vi "2-ReadAllFiles.vi"(8 "error in (no error)":errorcluster, 11 "AllControls IN":T1) -> (0 "error out":errorcluster, 3 "AllControls Out":T1)   [LabVIEW 2017]
uses:
  Ctrls/AllControls.ctl
  <vilib>/Utility/miscctls.llb/LVRowAndColumnTypeDef.ctl
  Ctrls/Position Config.ctl
  Ctrls/TesterInfo.ctl
  Ctrls/HD Config.ctl
  <vilib>/Utility/file.llb/Read Delimited Spreadsheet (string).vi
  ComVIS/Files/Ini/ReadIniFiles_ByVarient.vi
  <vilib>/regexp/Match Regular Expression.xnode
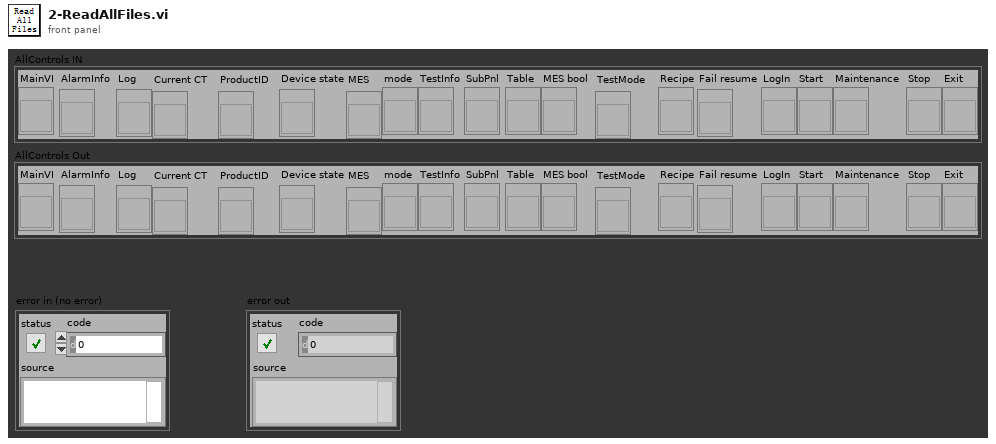
[diagram p1: front panel]
types:
  T1 = typedef "AllControls.ctl" = cluster{"MainVI":refnum<vi>, "AlarmInfo":refnum<vi>, "Log":refnum<vi>, "Current CT":refnum<vi>, "ProductID":refnum<vi>, "Device state":refnum<vi>, "MES":refnum<vi>, "mode":refnum<vi>, "TestInfo":refnum<vi>, "SubPnl":refnum<vi>, "Table":refnum<vi>, "MES bool":refnum<vi>, "TestMode":refnum<vi>, "Recipe":refnum<vi>, "Fail resume":refnum<vi>, "LogIn":refnum<vi>, "Start":refnum<vi>, "Maintenance":refnum<vi>, "Stop":refnum<vi>, "Exit":refnum<vi>}
  T2 = typedef "HD Config.ctl" = cluster{" PC":cluster{"PC Address":u8[], "PC Port":i32}, "FCO":cluster{"COM":refnum<visa-resource-name>, "Baudrate":u32}, "DC Power ":cluster{"COM":refnum<visa-resource-name>, "Baudrate":u32}, "PW3336":cluster{"COM":refnum<visa-resource-name>, "Baudrate":u32}, "Lefoo":cluster{"COM":refnum<visa-resource-name>, "Baudrate":u32}, "Tempt&Hum":cluster{"COM":refnum<visa-resource-name>, "Baudrate":u32}, "DIPC":cluster{"COM":refnum<visa-resource-name>}, "Daemon":cluster{"IP Address":string, "Port":u16, "Retry":u16}, "NFC_Cmd":cluster{"COM":refnum<visa-resource-name>, "Baudrate":u32}, "Fail_resume_mode":bool, "GRR":bool, "NFC _Serial":cluster{"COM":refnum<visa-resource-name>, "Baudrate":u32}}
  T3 = typedef "TesterInfo.ctl" = cluster{"Station Name":string, "Station Code":string, "ES NO.":string, "Tester ID":string, "PassMark Revision":string, "Rig ID":string, "682_Tool_Repeat":string, "Project Name":string, "FFTesterPath":path, "Enable_User":bool, "Mode":enum16{"682"}, "Fail_resume_mode":bool}
  T4 = typedef "Position Config.ctl" = cluster{"Black":dbl, "White":dbl, "Black1":dbl, "White1":dbl}
  T5 = typedef "LVRowAndColumnTypeDef.ctl" = cluster{"Row":i32, "Column":i32}
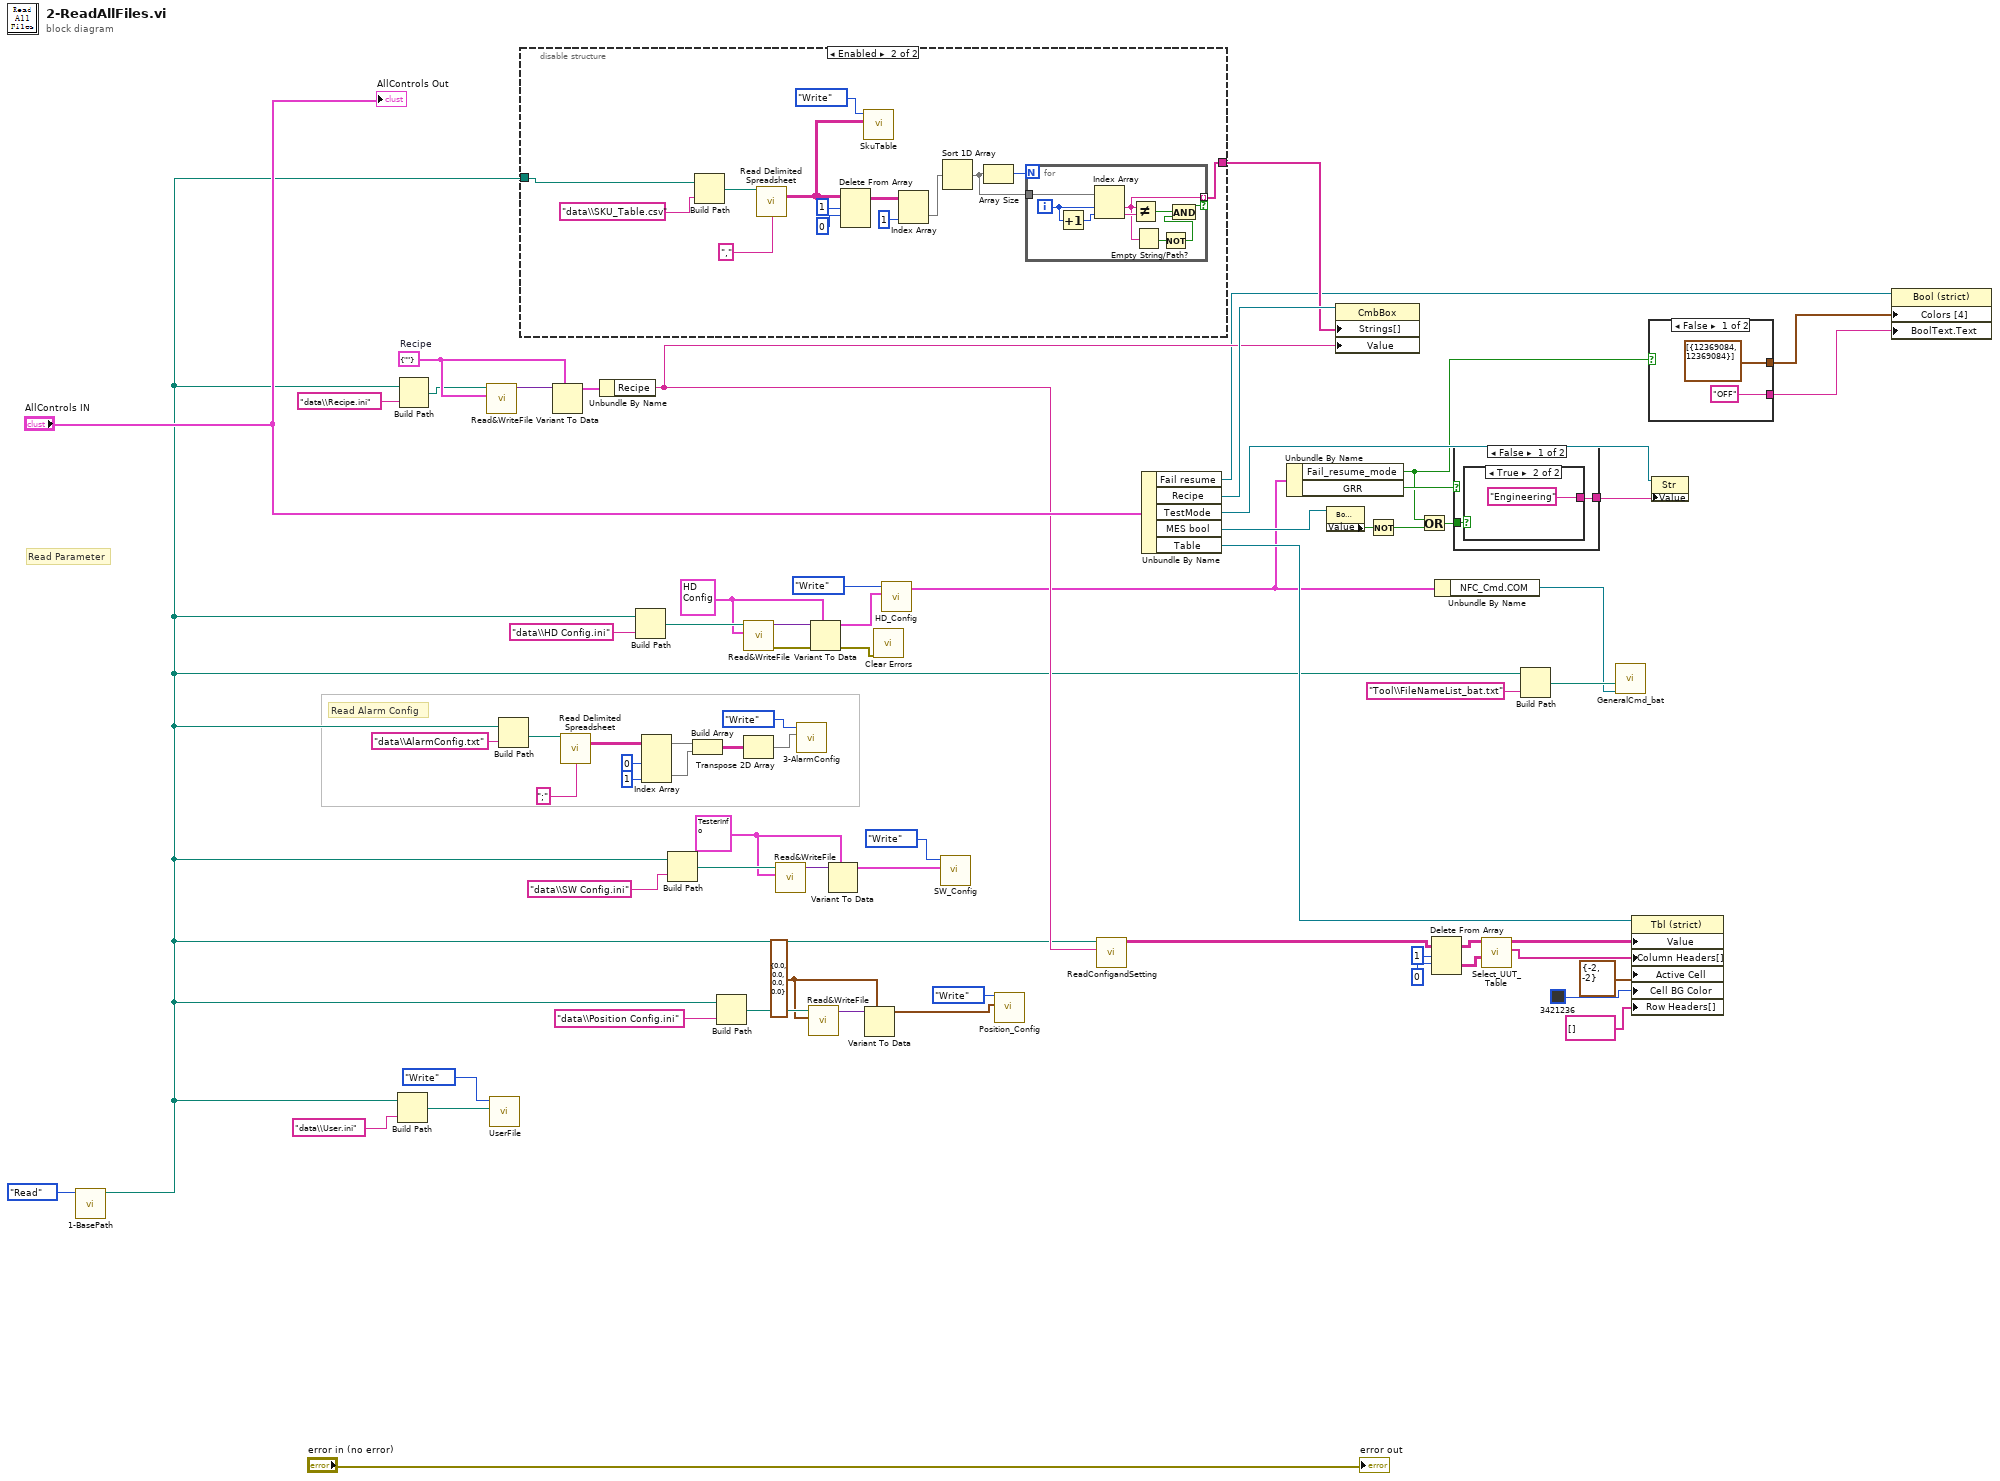
[diagram p0: block diagram]
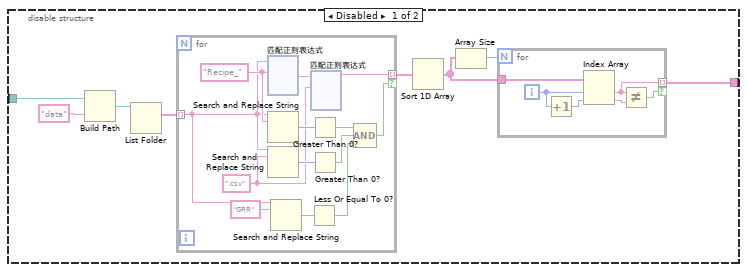
[diagram p2: hidden frame]
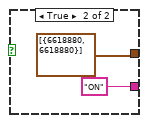
[diagram p3: hidden frame]
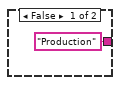
[diagram p4: hidden frame]
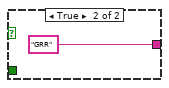
[diagram p5: hidden frame]
diagram:
  w15 = cluster{"Recipe":string} {"Recipe"=""}  # Recipe
  w26 = T2 {" PC"={"PC Address"=[], "PC Port"=0}, "FCO"={"COM"="", "Baudrate"=0}, "DC Power "={"COM"="", "Baudrate"=0}, "PW3336"={"COM"="", "Baudrate"=0}, "Lefoo"={"COM"="", "Baudrate"=0}, "Tempt&Hum"={"COM"="", "Baudrate"=0}, "DIPC"={"COM"=""}, "Daemon"={"IP Address"="", "Port"=0, "Retry"=0}, "NFC_Cmd"={"COM"="", "Baudrate"=0}, "Fail_resume_mode"=FALSE, "GRR"=FALSE, "NFC _Serial"={"COM"="", "Baudrate"=0}} ("HD Config")
  w27 = T3 {"Station Name"="", "Station Code"="", "ES NO."="", "Tester ID"="", "PassMark Revision"="", "Rig ID"="", "682_Tool_Repeat"="", "Project Name"="", "FFTesterPath"=path "", "Enable_User"=FALSE, "Mode"=enum."682", "Fail_resume_mode"=FALSE} ("TesterInfo")
  w30 = T4 {"Black"=0.0, "White"=0.0, "Black1"=0.0, "White1"=0.0} ("Position Config")
  # "Read Alarm Config"
  # "Read Parameter"
  n1 = call "1-BasePath.vi"("Step"=enum16{"Initial", "Write", "Read"}."Read") -> ("Path Out"=w1:path)  [unwired: 9 in, 1 out]
  n2 = Build Path(base path=w1, name or relative path="data\\User.ini") -> (appended path=w48:path)
  n3 = Build Path(base path=w1, name or relative path="data\\Recipe.ini") -> (appended path=w12:path)
  n4 = call-poly "Read&WriteFile.vi"("Varient"=w15, "path"=w12) -> ("DataOut"=w16:variant)  [unwired: 8 in, 1 out]
  n5 = call "UserFile.vi"("UserPath in"=w48, "Step"=enum16{"Initial", "Write", "Read"}."Write") -> ()  [unwired: 8 in, 2 out]
  n6 = Build Path(base path=w1, name or relative path="data\\AlarmConfig.txt") -> (appended path=w63:path)
  n7 = disable-structure shown="Enabled" {
    disable-tunnel: [w74 w330] -> w17
    disable-tunnel: w1 -> [w73 w337]
    frame Disabled {
      n8 = Build Path(base path=w73, name or relative path="data") -> (appended path=w79:path)
      n9 = List Folder(path=w79) -> (filenames=w78:string[])  [unwired: 3 in, 3 out]
      n10 = for {
        tunnel: w78 -> [w90] mode=indexing
        tunnel: [w91] -> w77 mode=indexing if=w97
        w92 = ".csv" ("搜索字符串")
        w94 = "Recipe_" ("搜索字符串")
        n11 = xnode "匹配正则表达式"("输入字符串"=w90, "正则表达式"=w94) -> ("匹配之后"=w93:string)  [unwired: 4 in, 4 out]
        n12 = Search and Replace String(input string=w90, search string=w94) -> (number of replacements=w99:i32)  [unwired: 6 in, 3 out]
        n13 = Search and Replace String(input string=w90, search string=w92) -> (number of replacements=w96:i32)  [unwired: 6 in, 3 out]
        n14 = Search and Replace String(input string=w90, search string="GRR" ("搜索字符串")) -> (number of replacements=w88:i32)  [unwired: 6 in, 3 out]
        n15 = Less Or Equal To 0?(x=w88) -> (x <= 0?=w87:bool)
        n16 = Greater Than 0?(x=w99) -> (x > 0?=w98:bool)
        n17 = Greater Than 0?(x=w96) -> (x > 0?=w95:bool)
        n18 = xnode "匹配正则表达式"("输入字符串"=w93, "正则表达式"=w92) -> ("匹配之前"=w91:string)  [unwired: 4 in, 4 out]
        n19 = Compound Arithmetic op=AND ("复合运算")(w98, w95, w87) -> (w97:bool)
      }
      n20 = Sort 1D Array(array=w77) -> (sorted array=w75:string[])
      n21 = Array Size(array=w75) -> (size(s)=w76:i32)
      n22 = for {
        N: w76 -> [_]
        tunnel: w75 -> [w86]
        tunnel: [w82] -> w74 mode=indexing if=w85
        i -> [w84]
        n23 = Increment(x=w84) -> (x+1=w83:i32)
        n24 = Index Array(array=w86, index #1=w84, index #2=w83) -> (element #1=w82:string, element #2=w81:string)
        n25 = Not Equal?(x=w82, y=w81) -> (x != y?=w85:bool)
      }
    }
    frame Enabled {
      n26 = Build Path(base path=w337, name or relative path="data\\SKU_Table.csv") -> (appended path=w341:path)
      n27 = call-poly <vilib>:"Read Delimited Spreadsheet.vi"("file path (dialog if empty)"=w341, "delimiter (\\t)"="," ("delimiter (\\t)")) -> ("all rows"=w336:string[][])  [unwired: 8 in, 5 out]
      n28 = Delete From Array(array=w336, length=1 ("长度"), index (row)=0 ("索引 (行)")) -> (array with subset deleted=w333:string[][])  [unwired: 1 in, 1 out]
      n29 = call "SkuTable.vi"("Tabledata in"=w336, "Step"=enum16{"Initial", "Write", "Read"}."Write") -> ()  [unwired: 8 in, 2 out]
      n30 = Index Array(array=w333, index (col)=1 ("禁用的索引 (列)")) -> (element=w328:string[])  [unwired: 1 in]
      n31 = Sort 1D Array(array=w328) -> (sorted array=w329:string[])
      n32 = Array Size(array=w329) -> (size(s)=w331:i32)
      n33 = for {
        N: w331 -> [_]
        tunnel: w329 -> [w350]
        tunnel: [w345] -> w330 mode=indexing if=w343
        i -> [w348]
        n34 = Increment(x=w348) -> (x+1=w347:i32)
        n35 = Index Array(array=w350, index #1=w348, index #2=w347) -> (element #1=w345:string, element #2=w346:string)
        n36 = Not Equal?(x=w345, y=w346) -> (x != y?=w349:bool)
        n37 = Empty String/Path?(string/path=w345) -> (empty?=w344:bool)
        n38 = Not(x=w344) -> (.not. x?=w342:bool)
        n39 = And(x=w349, y=w342) -> (x .and. y?=w343:bool)
      }
    }
  }
  n40 = Variant To Data(type=w15, Variant=w16) -> (data=w14:cluster{"Recipe":string})  [unwired: 1 in, 1 out]
  n41 = call-poly <vilib>:"Read Delimited Spreadsheet.vi"("file path (dialog if empty)"=w63, "delimiter (\\t)"=";" ("delimiter (\\t)")) -> ("all rows"=w60:string[][])  [unwired: 8 in, 5 out]
  n42 = Unbundle By Name(w14) -> ("Recipe"=w11:string)
  n43 = Build Path(base path=w1, name or relative path="data\\HD Config.ini") -> (appended path=w68:path)
  n44 = Index Array(array=w60, index (col) #1=0 ("disabled index (col)"), index (col) #2=1 ("index (col)")) -> (element #1=w59:string[], element #2=w55:string[])  [unwired: 2 in]
  n45 = Build Path(base path=w1, name or relative path="data\\SW Config.ini") -> (appended path=w52:path)
  n46 = Build Array(w59, w55) -> (w56:string[][])
  n47 = Build Path(base path=w1, name or relative path="data\\Position Config.ini") -> (appended path=w33:path)
  n48 = call-poly "Read&WriteFile.vi"("Varient"=w26, "path"=w68) -> ("error out"=w66:errorcluster, "DataOut"=w67:variant)  [unwired: 8 in]
  n49 = Transpose 2D Array(2D array=w56) -> (transposed array=w54:string[][])
  n50 = call-poly "Read&WriteFile.vi"("Varient"=w27, "path"=w52) -> ("DataOut"=w50:variant)  [unwired: 8 in, 1 out]
  n51 = call "3-AlarmConfig.vi"("AlarmConfig In"=w54, "Step"=enum16{"Initial", "Write", "Read"}."Write") -> ()  [unwired: 8 in, 2 out]
  n52 = call-poly "Read&WriteFile.vi"("Varient"=w30, "path"=w33) -> ("DataOut"=w31:variant)  [unwired: 8 in, 1 out]
  n53 = Variant To Data(error in=w66, type=w26, Variant=w67) -> (data=w46:T2, error out=w65:errorcluster)
  n54 = Variant To Data(type=w27, Variant=w50) -> (data=w45:T3)  [unwired: 1 in, 1 out]
  n55 = Variant To Data(type=w30, Variant=w31) -> (data=w29:T4)  [unwired: 1 in, 1 out]
  n56 = call <vilib>:"Clear Errors.vi"("error in (no error)"=w65) -> ()  [unwired: 5 in, 2 out]
  n57 = call "HD_Config.vi"("HD Config in"=w46, "Step"=enum16{"Initial", "Write", "Read"}."Write") -> ("HD Config out"=w2:T2)  [unwired: 8 in, 1 out]
  n58 = call "SW_Config.vi"("SW Config In"=w45, "Step"=enum16{"Initial", "Write", "Read"}."Write") -> ()  [unwired: 8 in, 2 out]
  n59 = call "Position_Config.vi"("Position Config"=w29, "Step"=enum16{"Initial", "Write", "Read"}."Write") -> ()  [unwired: 8 in, 2 out]
  n60 = call "ReadConfigandSetting.vi"("Recipe"=w11, "Path Out"=w1) -> ("TableData"=w37:string[][])  [unwired: 7 in, 2 out]
  n61 = Unbundle By Name("AllControls IN") -> ("Fail resume"=w8:refnum<vi>, "Recipe"=w18:refnum<vi>, "TestMode"=w23:refnum<vi>, "MES bool"=w24:refnum<vi>, "Table"=w39:refnum<vi>)
  n62 = Unbundle By Name(w2) -> ("Fail_resume_mode"=w9:bool, "GRR"=w25:bool)
  n63 = property class="Bool (严格)"(reference=w24) -> ("Value"=w21:bool)  [unwired: 1 in, 2 out]
  n64 = property class="CmbBox"(reference=w18, "Strings[]"=w17, "Value"=w11) -> ()  [unwired: 1 in, 2 out]
  n65 = Not(x=w21) -> (.not. x?=w19:bool)
  n66 = Or(x=w9, y=w19) -> (x .or. y?=w20:bool)
  n67 = Delete From Array(array=w37, length=1 ("长度"), index (row)=0 ("索引 (行)")) -> (deleted portion=w35:string[][], array with subset deleted=w38:string[][])  [unwired: 1 in]
  n68 = Unbundle By Name(w2) -> ("NFC_Cmd.COM"=w3:refnum<visa-resource-name>)
  n69 = case shown="False" w25 {
    tunnel: w20 -> [w352 _]
    tunnel: [w351 "GRR"] -> w22
    frame False {
      n70 = case shown="True" w352 {
        tunnel: ["Production" "Engineering"] -> w351
        frame False {
        }
        frame True {
        }
      }
    }
    frame True {
    }
  }
  n71 = call "Select_UUT_Table.vi"("all Title"=w35, "all Table"=w38) -> ("Title"=w36:string[], "Table"=w10:string[][])  [unwired: 8 in]
  n72 = Build Path(base path=w1, name or relative path="Tool\\FileNameList_bat.txt") -> (appended path=w4:path)
  n73 = call "GeneralCmd_bat.vi"("COM"=w3, "fileList_bat"=w4) -> ()  [unwired: 9 in, 1 out]
  n74 = property class="Tbl (strict)"(reference=w39, "Value"=w10, "Column Headers[]"=w36, "Active Cell"=T5 {"Row"=-2, "Column"=-2} ("活动单元格:活动单元格"), "Cell BG Color"=u32 3421236, "Row Headers[]"=string[] [] ("Row Header Strings[]")) -> ()  [unwired: 1 in, 2 out]
  n75 = case shown="False" w9 {
    tunnel: [cluster{u32, u32}[] [{12369084, 12369084}] cluster{u32, u32}[] [{6618880, 6618880}]] -> w7
    tunnel: ["OFF" "ON"] -> w6
    frame False {
    }
    frame True {
    }
  }
  n76 = property class="Str"(reference=w23, "Value"=w22) -> ()  [unwired: 1 in, 2 out]
  n77 = property on="属性节点" class="Bool (strict)"(reference=w8, "Colors [4]"=w7, "BoolText.Text"=w6) -> ()  [unwired: 1 in, 2 out]
  "AllControls Out" <- "AllControls IN"
  "error out" <- "error in (no error)"
